vi "SetAttributeViReal64.vi"(7 "AttributeValue":dbl, 8 "error in (no error)":errorcluster {"code" format="%.0x"}, 9 "AttributeID":u32(ring)=1150004 items=["CHANNEL_CW_FREQUENCY"=1150004, "CHANNEL_IF_BANDWIDTH"=1150005, "CHANNEL_MEASUREMENT_ELECTRICAL_DELAY_DISTANCE"=1150177, "CHANNEL_MEASUREMENT_ELECTRICAL_DELAY_TIME"=1150176, "CHANNEL_MEASUREMENT_ELECTRICAL_DELAY_VELOCITY_FACTOR"=1150180, "CHANNEL_MEASUREMENT_ELECTRICAL_DELAY_WAVE_GUIDE_CUT_OFF_FREQ"=1150179, "CHANNEL_MEASUREMENT_GROUP_DELAY_FREQUENCY"=1150172, "CHANNEL_MEASUREMENT_GROUP_DELAY_PERCENT"=1150174, "CHANNEL_MEASUREMENT_GROUP_DELAY_POINTS"=1150173, "CHANNEL_MEASUREMENT_MARKER_BANDWIDTH_THRESHOLD"=1150021, "CHANNEL_MEASUREMENT_MARKER_PEAK_EXCURSION"=1150024, "CHANNEL_MEASUREMENT_MARKER_STIMULUS"=1150025, "CHANNEL_MEASUREMENT_MARKER_TARGET_VALUE"=1150026, "CHANNEL_MEASUREMENT_SMOOTHING_APERTURE"=1150016, "CHANNEL_MEASUREMENT_TIME_DOMAIN_GATING_CENTER"=1150138, "CHANNEL_MEASUREMENT_TIME_DOMAIN_GATING_SPAN"=1150141, "CHANNEL_MEASUREMENT_TIME_DOMAIN_GATING_START"=1150142, "CHANNEL_MEASUREMENT_TIME_DOMAIN_GATING_STOP"=1150143, "CHANNEL_MEASUREMENT_TIME_DOMAIN_TRANSFORM_CENTER"=1150145, "CHANNEL_MEASUREMENT_TIME_DOMAIN_TRANSFORM_SPAN"=1150148, "CHANNEL_MEASUREMENT_TIME_DOMAIN_TRANSFORM_START"=1150149, "CHANNEL_MEASUREMENT_TIME_DOMAIN_TRANSFORM_STEP_RISE_TIME"=1150150, "CHANNEL_MEASUREMENT_TIME_DOMAIN_TRANSFORM_STOP"=1150151, "CHANNEL_MEASUREMENT_TIME_DOMAIN_WINDOW_IMPULSE_WIDTH"=1150152, "CHANNEL_MEASUREMENT_TIME_DOMAIN_WINDOW_KAISER_BETA"=1150153, "CHANNEL_MEASUREMENT_TRACE_REFERENCE_POSITION"=1150027, "CHANNEL_MEASUREMENT_TRACE_REFERENCE_VALUE"=1150028, "CHANNEL_MEASUREMENT_TRACE_Y_SCALE"=1150029, "CHANNEL_STIMULUS_RANGE_CENTER"=1150032, "CHANNEL_STIMULUS_RANGE_SPAN"=1150033, "CHANNEL_STIMULUS_RANGE_START"=1150034, "CHANNEL_STIMULUS_RANGE_STOP"=1150035, "CHANNEL_SWEEP_TIME"=1150010, "GUIDED_CALIBRATION__ADVANCED_IF_BAND_WIDTH"=1150171], 10 "RepCapIdentifier":string, 11 "instrument handle":refnum<k15>) -> (0 "error out":errorcluster {"code" format="%.0x"}, 3 "instrument handle out":refnum<k15>)   [LabVIEW 2014, in "Agilent NA.lvlib"]
doc: "Sets a Real64 attribute from the instrument driver.\nThe following Attributes are supported:\n\nCHANNEL_CW_FREQUENCY\nCHANNEL_IF_BANDWIDTH\nCHANNEL_MEASUREMENT_ELECTRICAL_DELAY_DISTANCE\nCHANNEL_MEASUREMENT_ELECTRICAL_DELAY_TIME\nCHANNEL_MEASUREMENT_ELECTRICAL_DELAY_VELOCITY_FACTOR\nCHANNEL_MEASUREMENT_ELECTRICAL_DELAY_WAVE_GUIDE_CUT_OFF_FREQ\nCHANNEL_MEASUREMENT_GROUP_DELAY_FREQUENCY\nCHANNEL_MEASUREMENT_GROUP_DELAY_PERCENT\nCHANNEL_MEASUREMENT_GROUP_DELAY_POINTS\nCHANNEL_MEASUREMENT_MARKER_BANDWIDTH_THRESHOLD\nCHANNEL_MEASUREMENT_MARKER_PEAK_EXCURSION\nCHANNEL_MEASUREMENT_MARKER_STIMULUS\nCHANNEL_MEASUREMENT_MARKER_TARGET_VALUE\nCHANNEL_MEASUREMENT_SMOOTHING_APERTURE\nCHANNEL_MEASUREMENT_TIME_DOMAIN_GATING_CENTER\nCHANNEL_MEASUREMENT_TIME_DOMAIN_GATING_SPAN\nCHANNEL_MEASUREMENT_TIME_DOMAIN_GATING_START\nCHANNEL_MEASUREMENT_TIME_DOMAIN_GATING_STOP\nCHANNEL_MEASUREMENT_TIME_DOMAIN_TRANSFORM_CENTER\nCHANNEL_MEASUREMENT_TIME_DOMAIN_TRANSFORM_SPAN\nCHANNEL_MEASUREMENT_TIME_DOMAIN_TRANSFORM_START\nCHANNEL_MEASUREMENT_TIME_DOMAIN_TRANSFORM_STEP_RISE_TIME\nCHANNEL_MEASUREMENT_TIME_DOMAIN_TRANSFORM_STOP\nCHANNEL_MEASUREMENT_TIME_DOMAIN_WINDOW_IMPULSE_WIDTH\nCHANNEL_MEASUREMENT_TIME_DOMAIN_WINDOW_KAISER_BETA\nCHANNEL_MEASUREMENT_TRACE_REFERENCE_POSITION\nCHANNEL_MEASUREMENT_TRACE_REFERENCE_VALUE\nCHANNEL_MEASUREMENT_TRACE_Y_SCALE\nCHANNEL_STIMULUS_RANGE_CENTER\nCHANNEL_STIMULUS_RANGE_SPAN\nCHANNEL_STIMULUS_RANGE_START\nCHANNEL_STIMULUS_RANGE_STOP\nCHANNEL_SWEEP_TIME\nGUIDED_CALIBRATION__ADVANCED_IF_BAND_WIDTH"
uses:
  Agilent NA.lvlib
  AgNA.dll
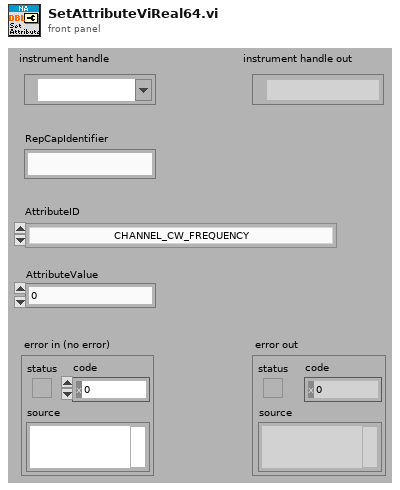
[diagram p1: front panel]
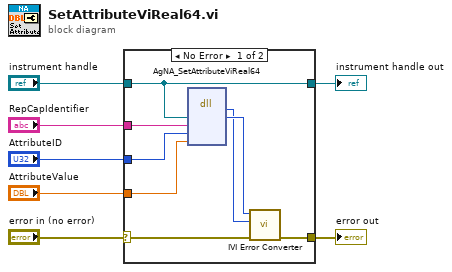
[diagram p0: block diagram]
diagram:
  n1 = case shown="No Error" "error in (no error)" {
    selector: "error in (no error)" -> [w13 w17]
    tunnel: [w12 w17] -> w7
    tunnel: "RepCapIdentifier" -> [w11 _]
    tunnel: "AttributeID" -> [w10 _]
    tunnel: "AttributeValue" -> [w9 _]
    tunnel: [w8 w16] -> w2
    tunnel: "instrument handle" -> [w8 w16]
    frame No Error {
      n2 = dll-call lib="AgNA**.dll" fn="AgNA_SetAttributeViReal64"("Vi"=w8, "RepCapIdentifier"=w11, "AttributeID"=w10, "AttributeValue"=w9) -> ("return type"=w14:i32, "Vi"=w15:u32)  [unwired: 6 in, 2 out]
      n3 = call "IVI Error Converter.vi"("error in (no error)"=w13, "IVI error code (0)"=w14, "instrument handle"=w15) -> ("error out"=w12:errorcluster)  [unwired: 7 in, 1 out]
    }
    frame Error {
    }
  }
  "error out" <- w7
  "instrument handle out" <- w2
